vi "selectColor.vi"() -> (2 "ok":bool, 3 "Color out":u32(colorbox))   [LabVIEW 2017, in "QControl_Graph.lvclass"]
uses:
  QControl_Graph.lvclass
panel:
  in  "Color":u32(colorbox)
  in  "Cancel":bool
  in  "OK":bool
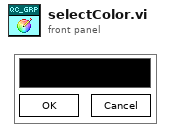
[diagram p1: front panel]
types:
  T1 = enum32{"Invalid", "Standard", "Closed", "Hidden", "Minimized", "Maximized"}
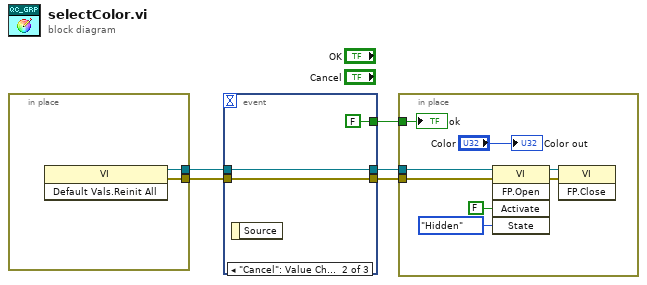
[diagram p0: block diagram]
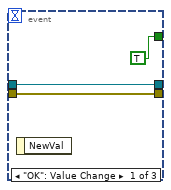
[diagram p2: hidden frame]
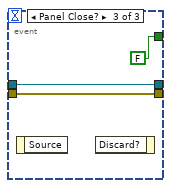
[diagram p3: hidden frame]
diagram:
  n1 = in-place {
    in-place-border: [w7] -> w3
    in-place-border: [w6] -> w2
    n2 = invoke class="VI" method="Default Vals.Reinit All"() -> (reference out=w6:refnum<vi>, error out=w7:errorcluster)  [unwired: 3 in, 1 out]
  }
  n3 = event shown="[1] \"Cancel\": Value Change" {
    selector: _ -> [_ _ _]
    dyn-events: _ -> [_ _ _]
    timeout: _ -> [_ _ _]
    tunnel: [TRUE FALSE FALSE] -> w5
    tunnel: w3 -> [w8 w12 w14]
    tunnel: [w8 w12 w14] -> w4
    tunnel: w2 -> [w9 w11 w15]
    tunnel: [w9 w11 w15] -> w1
    event "OK": Value Change {
      n4 = event-data() -> ()  [unwired: 1 in, 1 out]
    }
    event "Cancel": Value Change {
      n5 = event-data() -> ()  [unwired: 1 in, 1 out]
    }
    event Panel Close? {
      n6 = event-data() -> ()  [unwired: 1 in, 1 out]
      n7 = event-data() -> ()  [unwired: 2 in, 1 out]
    }
  }
  n8 = in-place {
    in-place-border: w5 -> [w24]
    in-place-border: w4 -> [w18]
    in-place-border: w1 -> [w17]
    n9 = invoke class="VI" method="FP.Open"(reference=w17, error in=w18, "Activate"=FALSE ("Activate?"), "State"=T1."Hidden") -> (reference out=w23:refnum<vi>, error out=w22:errorcluster)  [unwired: 1 in, 3 out]
    n10 = invoke class="VI" method="FP.Close"(reference=w23, error in=w22) -> ()  [unwired: 1 in, 3 out]
    "ok" <- w24
    "Color out" <- "Color"
  }
